vi "create_resources.vi"(8 "error in (no error)":errorcluster) -> (0 "error out":errorcluster, 3 "Queues":T1)   [LabVIEW 2025, in "LabJackEKG.lvlib"]
uses:
  LabJackEKG.lvlib
  Typedefs/LabJackQueues.ctl
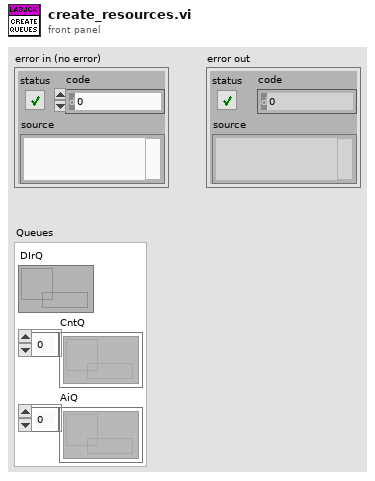
[diagram p1: front panel]
types:
  T1 = cluster{"DIrQ":refnum<queue>, "CntQ":refnum<queue>[], "AiQ":refnum<queue>[]}
  T2 = typedef "LabJackEKG.lvlib/LabJackQueues.ctl" = cluster{"DIrQ":refnum<queue>, "CntQ":refnum<queue>[], "AiQ":refnum<queue>[]}
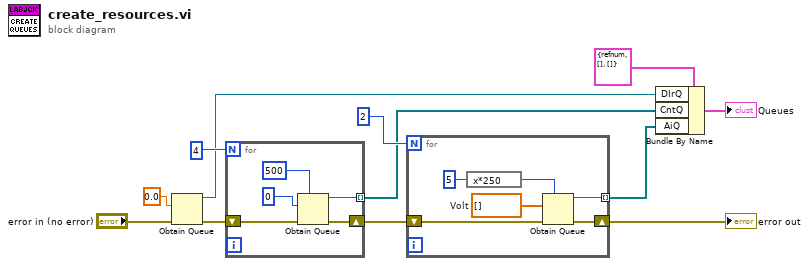
[diagram p0: block diagram]
diagram:
  n1 = Obtain Queue(element data type=0.0, error in (no error)="error in (no error)") -> (queue out=w3:refnum<queue>, error out=w8:errorcluster)  [unwired: 3 in, 1 out]
  n2 = for {
    N: 4 -> [_]
    tunnel: [w15] -> w2 mode=indexing
    shift-right: [w17] -> w7
    shift-left: w8 -> [w13]
    n3 = Obtain Queue(max queue size (-1, unlimited)=500, element data type=i64 0, error in (no error)=w13) -> (queue out=w15:refnum<queue>, error out=w17:errorcluster)  [unwired: 2 in, 1 out]
  }
  n4 = for {
    N: 2 -> [_]
    tunnel: [w22] -> w1 mode=indexing
    shift-right: [w19] -> w6
    shift-left: w7 -> [w18]
    w23 = dbl[] []  # Volt
    n5 = expression code="x*250"(5 ("max queue size (-1, unlimited)")) -> (w20:i32)
    n6 = Obtain Queue(max queue size (-1, unlimited)=w20, element data type=w23, error in (no error)=w18) -> (queue out=w22:refnum<queue>, error out=w19:errorcluster)  [unwired: 2 in, 1 out]
  }
  "error out" <- w6
  n7 = Bundle By Name(cluster=T2 {"DIrQ"=refnum, "CntQ"=[], "AiQ"=[]} ("Queues"), "DIrQ"=w3, "CntQ"=w2, "AiQ"=w1) -> (→"Queues":T2)
